vi "Configure CAN.vi"(8 "error in":errorcluster, 11 "HSU MCU V2 Monitor CFG in":refnum<class "HSU MCU V2 Monitor CFG.lvclass">) -> (0 "error out":errorcluster, 3 "HSU MCU V2 Monitor CFG out":refnum<class "HSU MCU V2 Monitor CFG.lvclass">)   [LabVIEW 2023, in "HSU MCU V2 Monitor CFG.lvclass"]
uses:
  HSU MCU V2 Monitor CFG.lvclass
  D:/git/HAL/HAL GOOP4/Configuration/Configuration JSON/Configuration JSON Base/CFG JSON.lvclass
  Configuration/Configuration JSON/Configuration JSON Base/CFG JSON.lvclass
  Protocols/ICAN/ICAN.lvclass
  Configuration/Configuration JSON/Configuration JSON Base/CFG JSON.lvclass/CFG JSON.ctl
  HSU MCU V2 Monitor CFG.lvclass/HSU MCU V2 Monitor CFG.ctl
  eac0ac60-99f7-48e2-bd7d-6d60fd840859.vi
  <vilib>/JDP Science/JSONtext/Next JSON Value.vi
  <vilib>/JDP Science/JSONtext/String Subset.vi
  <vilib>/JDP Science/JSONtext/Parsing/Advance past next JSON Value (inlined COPY).vi
  <vilib>/JDP Science/JSONtext/Parsing/Advance past whitespace.vi
  <vilib>/JDP Science/JSONtext/Parsing/Advance past String.vi
  <vilib>/JDP Science/JSONtext/Parsing/Advance past Number.vi
  <vilib>/JDP Science/JSONtext/Parsing/Advance past Line Ending.vi
  <vilib>/JDP Science/JSONtext/Parsing/Parse Full Path or Item Name.vi
  <vilib>/JDP Science/JSONtext/Parsing/Advance past Array.vi
  <vilib>/JDP Science/JSONtext/Parsing/Advance past Object.vi
  <vilib>/JDP Science/JSONtext/support/Error Cluster From Code.vi
  <vilib>/JDP Science/JSONtext/Offset/Find Item Locations by Path.vi
  <vilib>/JDP Science/JSONtext/JSON text to Variant.vi
  <vilib>/JDP Science/JSONtext/LVClass Serializer/JSONtext LVClass Serializer.lvclass
  <vilib>/JDP Science/JSONtext/JSONtext.lvlib
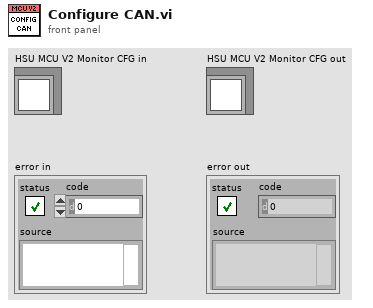
[diagram p1: front panel]
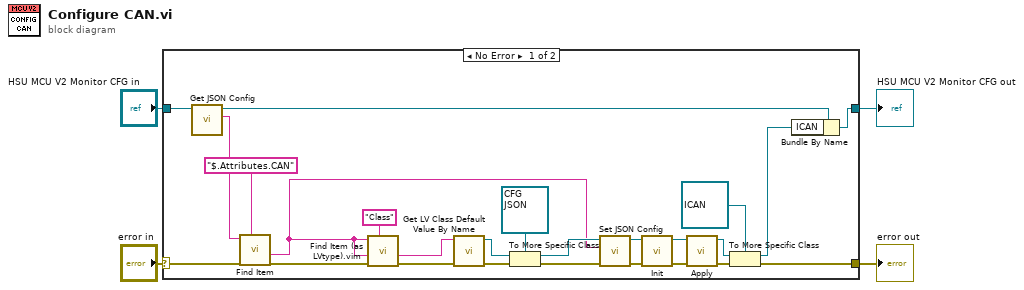
[diagram p0: block diagram]
diagram:
  n1 = case shown="No Error" "error in" {
    selector: "error in" -> [w23 w30]
    tunnel: [w15 w30] -> w3
    tunnel: [w26 w29] -> w1
    tunnel: "HSU MCU V2 Monitor CFG in" -> [w28 w29]
    frame No Error {
      n2 = call "Get JSON Config.vi"("CFG Base in"=w28) -> ("<JSON>Config>"=w7:string, "CFG Base out"=w27:refnum<class "HSU MCU V2 Monitor CFG.lvclass">)  [unwired: 9 in]
      n3 = call <vilib>:"Find Item.vi"("$Path or Item Name"="$.Attributes.CAN", "JSON"=w7) -> ("<JSON>"=w6:string)  [unwired: 6 in, 3 out]
      n4 = call "Find Item (as LVtype).vim"("$Path or Item Name"="Class", "error in (no error)"=w23, "Data Type and Default Value"=w6, "JSON"=w6) -> ("error out"=w24:errorcluster, "Data"=w5:string)  [unwired: 4 in, 2 out]
      n5 = call <vilib>:"Get LV Class Default Value By Name.vi"("error in (no error)"=w24, "class name"=w5) -> ("error out"=w25:errorcluster, "object"=w19:refnum<class>)  [unwired: 8 in]
      n6 = To More Specific Class(target class=refnum<class "CFG JSON.lvclass"> refnum ("ICommunicate.lvclass"), reference=w19, error in=w25) -> (specific class reference=w9:refnum<class "CFG JSON.lvclass">, error out=w21:errorcluster)
      n7 = call "Set JSON Config.vi"("error in (no error)"=w21, "<JSON>Config>"=w6, "CFG Base in"=w9) -> ("error out"=w11:errorcluster, "CFG Base out"=w10:refnum<class "CFG JSON.lvclass">)  [unwired: 7 in]
      n8 = call-dynamic "Init.vi"("error in"=w11, "IConfigure in"=w10) -> ("error out"=w18:errorcluster, "IConfigure out"=w16:refnum<class "CFG JSON.lvclass">)  [unwired: 8 in]
      n9 = call-dynamic "Apply.vi"("error in"=w18, "IConfigure in"=w16) -> ("error out"=w17:errorcluster, "IConfigure out"=w14:refnum<class "CFG JSON.lvclass">)  [unwired: 8 in]
      n10 = To More Specific Class(target class=refnum<class "ICAN.lvclass"> refnum ("ICAN.lvclass"), reference=w14, error in=w17) -> (specific class reference=w12:refnum<class "ICAN.lvclass">, error out=w15:errorcluster)
      n11 = Bundle By Name(cluster=w27, "ICAN"=w12) -> (w26:refnum<class "HSU MCU V2 Monitor CFG.lvclass">)
    }
    frame Error {
    }
  }
  "error out" <- w3
  "HSU MCU V2 Monitor CFG out" <- w1
